vi "ArrowHead_GetObjectStatus.vi"(0 "reference in":refnum<class "ArrowHead.lvclass">, 5 "error in (no error)":errorcluster) -> (14 "reference out":refnum<class "ArrowHead.lvclass">, 16 "Object name":string, 19 "error out":errorcluster)   [LabVIEW 2014, in "ArrowHead.lvclass"]
doc: "Returns the object status and also information about all the objects in the class.\n\n[GOOP 2.0.15]"
uses:
  <resource>/Framework/Providers/Open_GDS/UML/ArrowHead_class/ArrowHead.lvclass
  <resource>/Framework/Providers/Open_GDS/UML/ArrowHead_class/ArrowHead.lvclass/ArrowHead.ctl
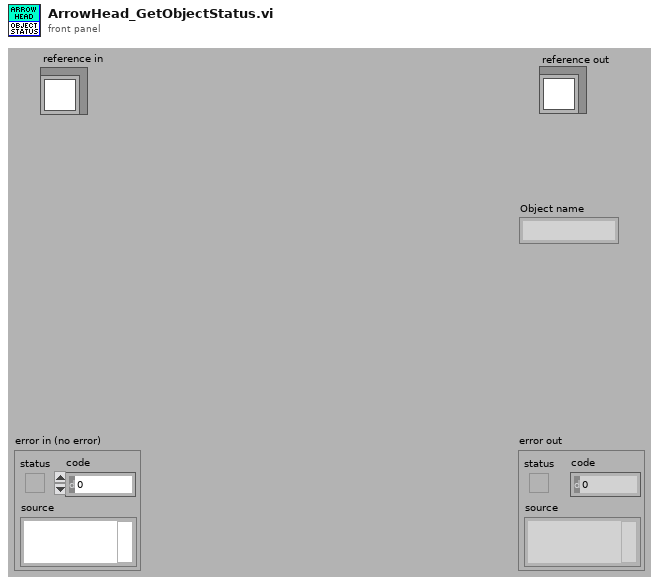
[diagram p1: front panel]
types:
  T1 = typedef "ArrowHead.lvclass/ArrowHeadType.ctl" = enum16{"NONE", "TRIANGLE", "BLACK_TRIANGLE", "V", "HALF_V", "DIAMOND", "BLACK_DIAMOND"}
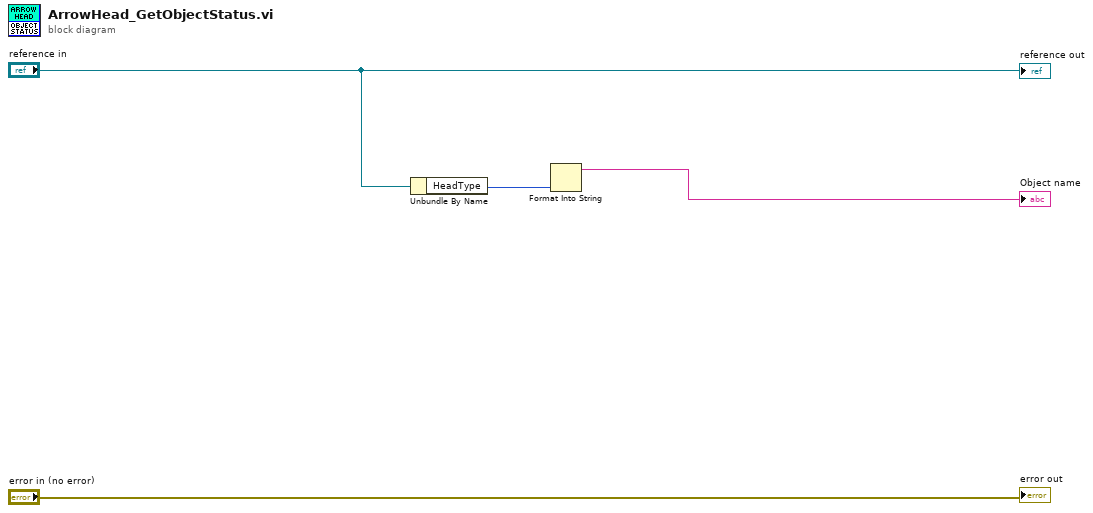
[diagram p0: block diagram]
diagram:
  n1 = Unbundle By Name("reference in") -> ("HeadType"=w3:T1)
  n2 = Format Into String(w3) -> (resulting string=→"Object name":string)  [unwired: 3 in, 1 out]
  "error out" <- "error in (no error)"
  "reference out" <- "reference in"
